vi "ep_Scaling Ratio (Single Line).vi"(8 "error in (no error)":errorcluster, 9 "system info in":refnum<class "EP System Info.lvclass">, 10 "CT/VT ratio":cluster{"primary":dbl, "secondary":dbl}[](array[cluster]), 11 "waveforms in":waveform(dbl)[](array[waveform])) -> (0 "error out":errorcluster, 1 "system info out":refnum<class "EP System Info.lvclass">, 3 "waveforms out":waveform(dbl)[](array[waveform]))   [LabVIEW 2014, in "NI_EP_Power Quality.lvlib"]
uses:
  <vilib>/addons/Electrical Power/PQ/NI_EP_Power Quality.lvlib
  <vilib>/addons/Electrical Power/PQ/Common/Classes/System Info/EP System Info.lvclass
  <vilib>/addons/Electrical Power/PQ/Common/Controls/ep_AI Data Channel.ctl
  <vilib>/addons/Electrical Power/PQ/Scaling_Calibration/subVIs/ep_Compute Third Current (DBL WFM).vi
panel:
  # ":"
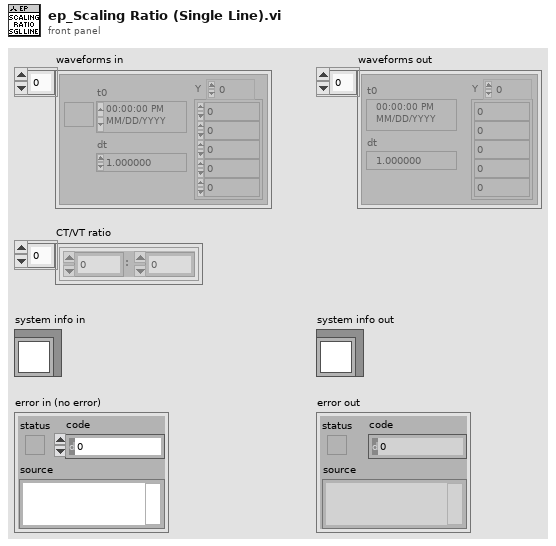
[diagram p1: front panel]
types:
  T1 = typedef "NI_EP_Power Quality.lvlib/ep_AI Data Channel.ctl" = enum16{"Voltage Phase A (L1)", "Voltage Phase B (L2)", "Voltage Phase C (L3)", "Voltage Phase N (Neutral)", "Current Phase A (L1)", "Current Phase B (L2)", "Current Phase C (L3)", "Current Phase N (Neutral)"}
  T2 = typedef "NI_EP_Power Quality.lvlib/ep_Wiring.ctl" = enum16{"4xUph + 4xI", "3xUph + 4xI", "3xUline + 4xI", "3xUph + 3xI", "3xUline + 3xI", "3xUph + 2xI", "3xUline + 2xI", "1xUph + 1xI"}
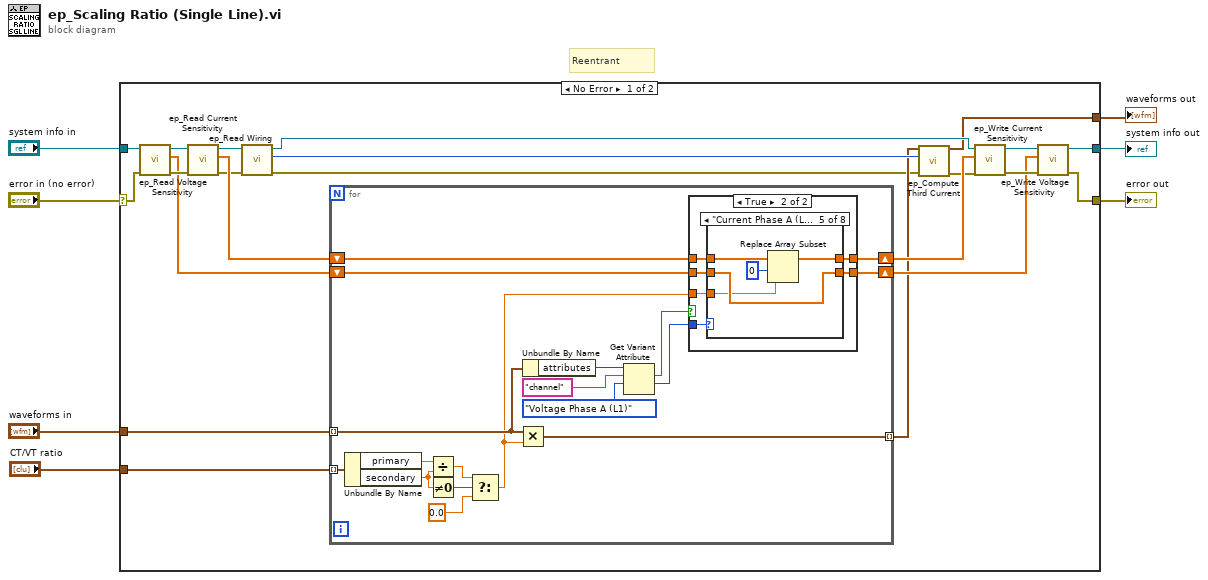
[diagram p0: block diagram]
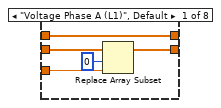
[diagram p3: hidden frame]
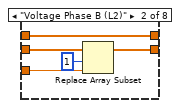
[diagram p4: hidden frame]
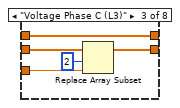
[diagram p5: hidden frame]
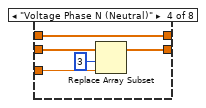
[diagram p6: hidden frame]
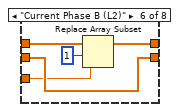
[diagram p7: hidden frame]
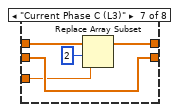
[diagram p8: hidden frame]
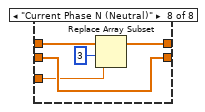
[diagram p9: hidden frame]
diagram:
  # "Reentrant"
  n1 = case shown="No Error" "error in (no error)" {
    selector: "error in (no error)" -> [w8 w96]
    tunnel: "waveforms in" -> [w14 _]
    tunnel: "CT/VT ratio" -> [w13 _]
    tunnel: "system info in" -> [w12 w97]
    tunnel: [w11 _] -> w4
    tunnel: [w10 w97] -> w3
    tunnel: [w9 w96] -> w2
    frame No Error {
      n2 = call <vilib>:"ep_Read Voltage Sensitivity.vi"("error in (no error)"=w8, "system info in"=w12) -> ("error out"=w28:errorcluster, "voltage sensitivity"=w27:dbl[], "system info out"=w29:refnum<class "EP System Info.lvclass">)  [unwired: 7 in]
      n3 = call <vilib>:"ep_Read Current Sensitivity.vi"("error in (no error)"=w28, "system info in"=w29) -> ("error out"=w18:errorcluster, "current sensitivity"=w26:dbl[], "system info out"=w20:refnum<class "EP System Info.lvclass">)  [unwired: 7 in]
      n4 = call <vilib>:"ep_Read Wiring.vi"("error in (no error)"=w18, "system info in"=w20) -> ("error out"=w15:errorcluster, "wiring"=w17:T2, "system info out"=w19:refnum<class "EP System Info.lvclass">)  [unwired: 6 in, 1 out]
      n5 = for {
        tunnel: w14 -> [w44] mode=indexing
        tunnel: w13 -> [w36] mode=indexing
        tunnel: [w47] -> w16 mode=indexing
        shift-right: [w41] -> w23
        shift-left: w26 -> [w43]
        shift-right: [w40] -> w21
        shift-left: w27 -> [w42]
        n6 = Unbundle By Name(w36) -> ("primary"=w37:dbl, "secondary"=w35:dbl)
        n7 = Divide(x=w37, y=w35) -> (x/y=w33:dbl)
        n8 = Not Equal To 0?(x=w35) -> (x != 0?=w34:bool)
        n9 = Select(t=w33, s=w34, f=0.0) -> (s? t:f=w31:dbl)
        n10 = Multiply(x=w44, y=w31) -> (x*y=w47:waveform(dbl))
        n11 = Unbundle By Name(w44) -> ("attributes"=w46:variant)
        n12 = Get Variant Attribute(Variant=w46, name="channel", default value (empty Variant)=ep_AI_Data_Channel."Voltage Phase A (L1)" ("AI data channel")) -> (found=w39:bool, value=w38:T1)  [unwired: 1 in, 2 out]
        n13 = case shown="True" w39 {
          tunnel: w38 -> [_ w55]
          tunnel: w31 -> [_ w54]
          tunnel: w42 -> [w49 w53]
          tunnel: [w49 w50] -> w40
          tunnel: [w48 w52] -> w41
          tunnel: w43 -> [w48 w51]
          frame False {
          }
          frame True {
            n14 = case shown="\"Current Phase A (L1)\"" w55 {
              tunnel: w54 -> [w59 w64 w69 w74 w76 w81 w86 w91]
              tunnel: w53 -> [w60 w65 w70 w75 w77 w82 w87 w92]
              tunnel: [w58 w63 w68 w73 w78 w83 w88 w93] -> w52
              tunnel: w51 -> [w58 w63 w68 w73 w79 w84 w89 w94]
              tunnel: [w57 w62 w67 w72 w77 w82 w87 w92] -> w50
              frame "Voltage Phase A (L1)", Default {
                n15 = Replace Array Subset(array=w60, new element=w59, index=0) -> (w57:dbl[])
              }
              frame "Voltage Phase B (L2)" {
                n16 = Replace Array Subset(array=w65, new element=w64, index=1) -> (w62:dbl[])
              }
              frame "Voltage Phase C (L3)" {
                n17 = Replace Array Subset(array=w70, new element=w69, index=2) -> (w67:dbl[])
              }
              frame "Voltage Phase N (Neutral)" {
                n18 = Replace Array Subset(array=w75, new element=w74, index=3) -> (w72:dbl[])
              }
              frame "Current Phase A (L1)" {
                n19 = Replace Array Subset(array=w79, new element=w76, index=0) -> (w78:dbl[])
              }
              frame "Current Phase B (L2)" {
                n20 = Replace Array Subset(array=w84, new element=w81, index=1) -> (w83:dbl[])
              }
              frame "Current Phase C (L3)" {
                n21 = Replace Array Subset(array=w89, new element=w86, index=2) -> (w88:dbl[])
              }
              frame "Current Phase N (Neutral)" {
                n22 = Replace Array Subset(array=w94, new element=w91, index=3) -> (w93:dbl[])
              }
            }
          }
        }
      }
      n23 = call-poly <vilib>:"ep_Compute Third Current.vi"("current waveforms in"=w16, "wiring"=w17, "error in (no error)"=w15) -> ("current waveforms out"=w11:waveform(dbl)[], "error out"=w22:errorcluster)  [unwired: 11 in]
      n24 = call <vilib>:"ep_Write Current Sensitivity.vi"("error in (no error)"=w22, "current sensitivity"=w23, "system info in"=w19) -> ("error out"=w25:errorcluster, "system info out"=w24:refnum<class "EP System Info.lvclass">)  [unwired: 7 in]
      n25 = call <vilib>:"ep_Write Voltage Sensitivity.vi"("error in (no error)"=w25, "voltage sensitivity"=w21, "system info in"=w24) -> ("error out"=w9:errorcluster, "system info out"=w10:refnum<class "EP System Info.lvclass">)  [unwired: 7 in]
    }
    frame Error {
    }
  }
  "error out" <- w2
  "waveforms out" <- w4
  "system info out" <- w3
